vi "loadSchedule.vi"() -> ()   [LabVIEW 2012]
uses:
  <vilib>/Utility/NIReport.llb/NI_report.lvclass
  <vilib>/addons/database/Auxilliary.llb/DB Tools Cursor Type.ctl
  <vilib>/addons/_office/_exclsub.llb/font.ctl
  <vilib>/addons/_office/excel.llb/Excel Get Data (str).vi
  <vilib>/addons/database/Connection.llb/DB Tools Open Connec (Path).vi
  <vilib>/addons/database/Connection.llb/Conn Execute.vi
  <vilib>/addons/database/Recordset.llb/Rec Fetch Recordset Data (R).vi
  <vilib>/addons/database/Recordset.llb/Rec Destroy - Connection.vi
  <vilib>/addons/database/_DB Variant To Data/Database Variant To Data.xnode
  <vilib>/Utility/NIReport.llb/Excel/NI_Excel.lvclass
  <vilib>/addons/_office/NI_ReportGenerationToolkit.lvlib
  <vilib>/addons/database/NI_Database_API.lvlib
panel:
  out "spreadsheet string":string
  in  "start (0, 0) 4":cluster{"start row":i32, "start column":i32}
  out "ExcelRow":i32
  out "output cluster":cluster{"start row":i32, "start column":i32}
  in  "start (0, 0) 3":cluster{"start row":i32, "start column":i32}
  out "concatenated string":string
  in  "template (empty) 2":path=path "O:/m100schedule/history/112199MT人力配置AT機台排程.xls"
  out "error out 4":errorcluster
  out "array":string[][](array[string])
  in  "start (0, 0) 2":cluster{"start row":i32, "start column":i32}
  out "data":string
  in  "template (empty)":path=path "O:/m100schedule/history/m100-schedule temp.xls"
  in  "start (0, 0)":cluster{"start row":i32, "start column":i32}
  out "x+y":i32
  out "row":i32
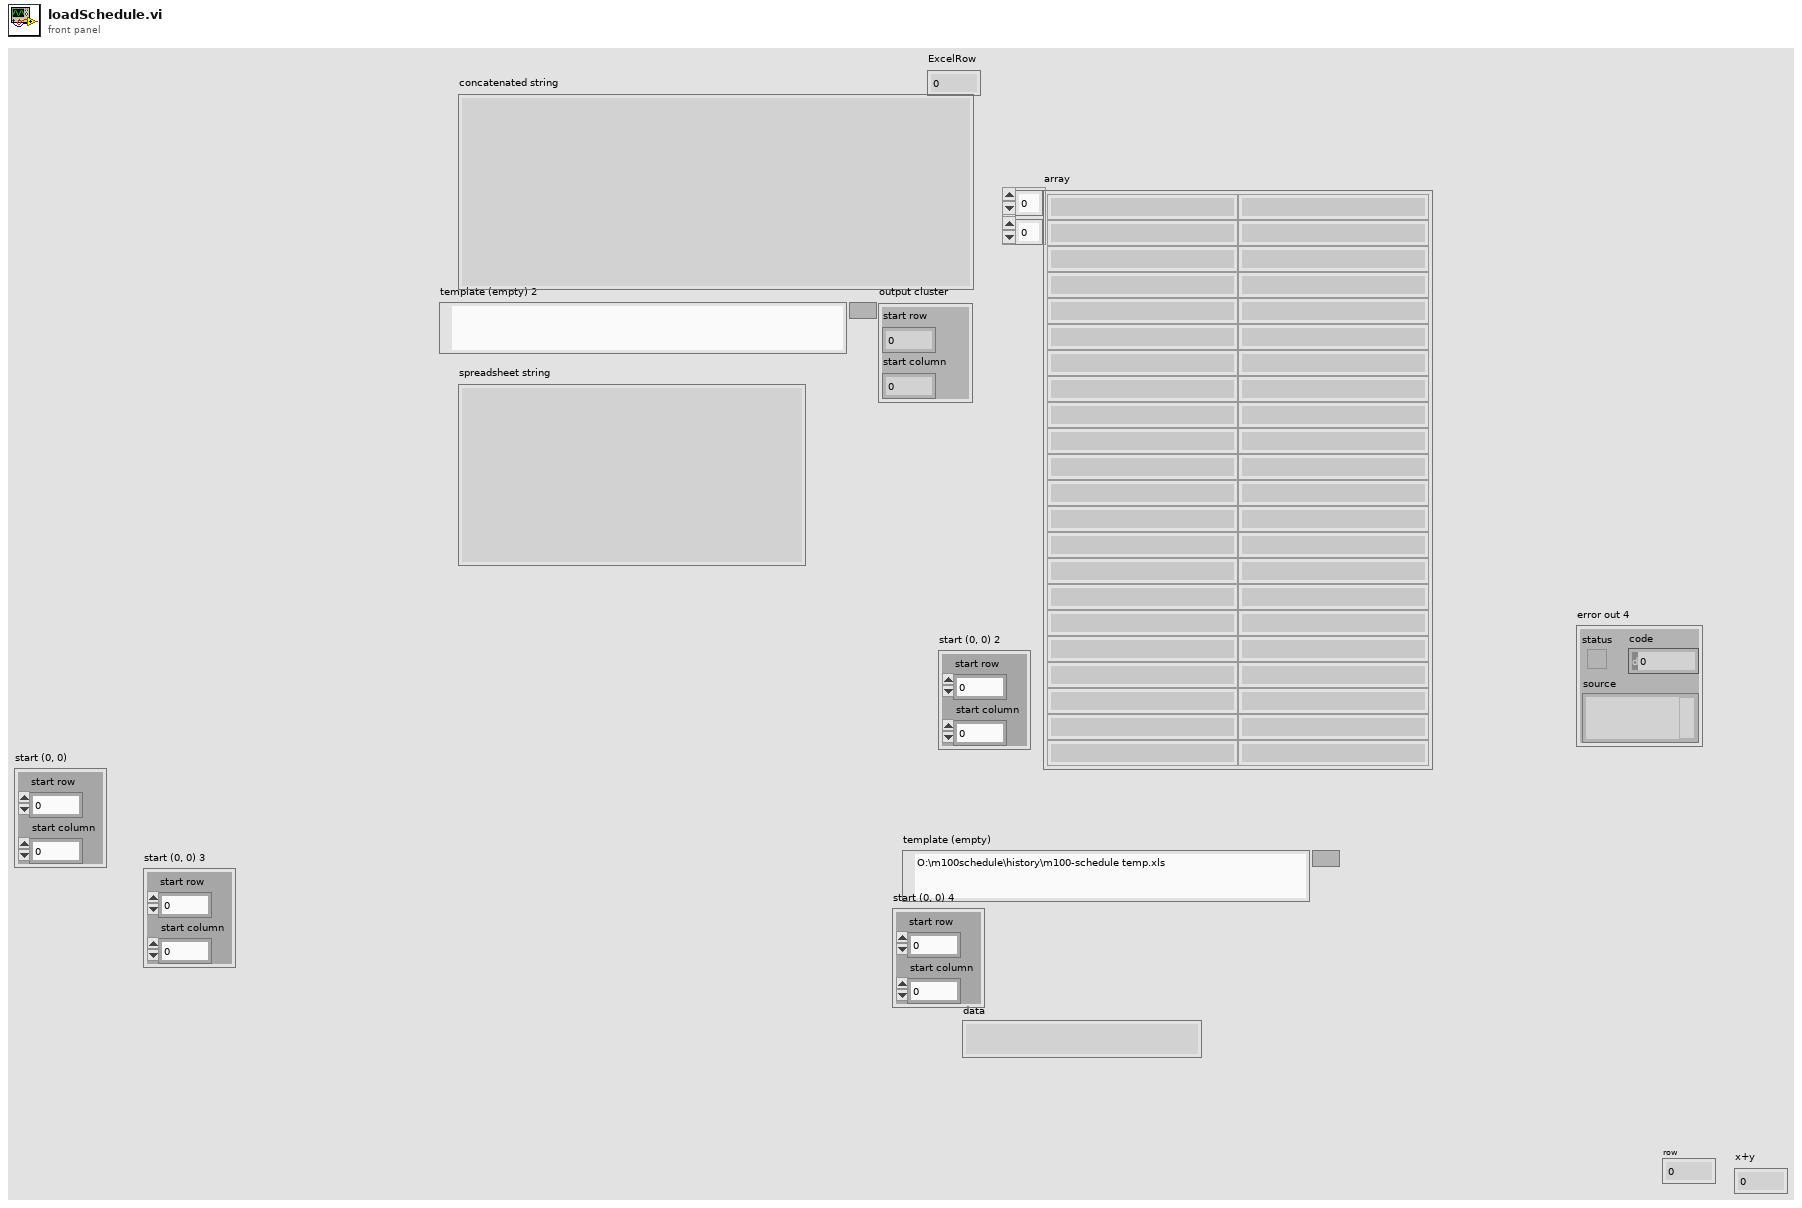
[diagram p1: front panel]
types:
  T1 = enum16{"Standard Report", "HTML", "Word", "Excel"}
  T2 = typedef "NI_Database_API.lvlib/DB Tools Cursor Type.ctl" = enum16{"forward-only", "keyset", "dynamic", "static"}
  T3 = typedef "NI_ReportGenerationToolkit.lvlib/font.ctl" = cluster{"font name":string, "font size":dbl, "bold":u16, "italic":u16, "underline":u16, "strike through":u16, "font color":u32}
  T4 = cluster{"on/off":bool, "weight":i32, "color":u32}
  T5 = typedef "NI_Database_API.lvlib/Conn ObjectReference.ctl" = refnum<k1>
  T6 = typedef "NI_Database_API.lvlib/Rec ObjectReference.ctl" = refnum<k1>
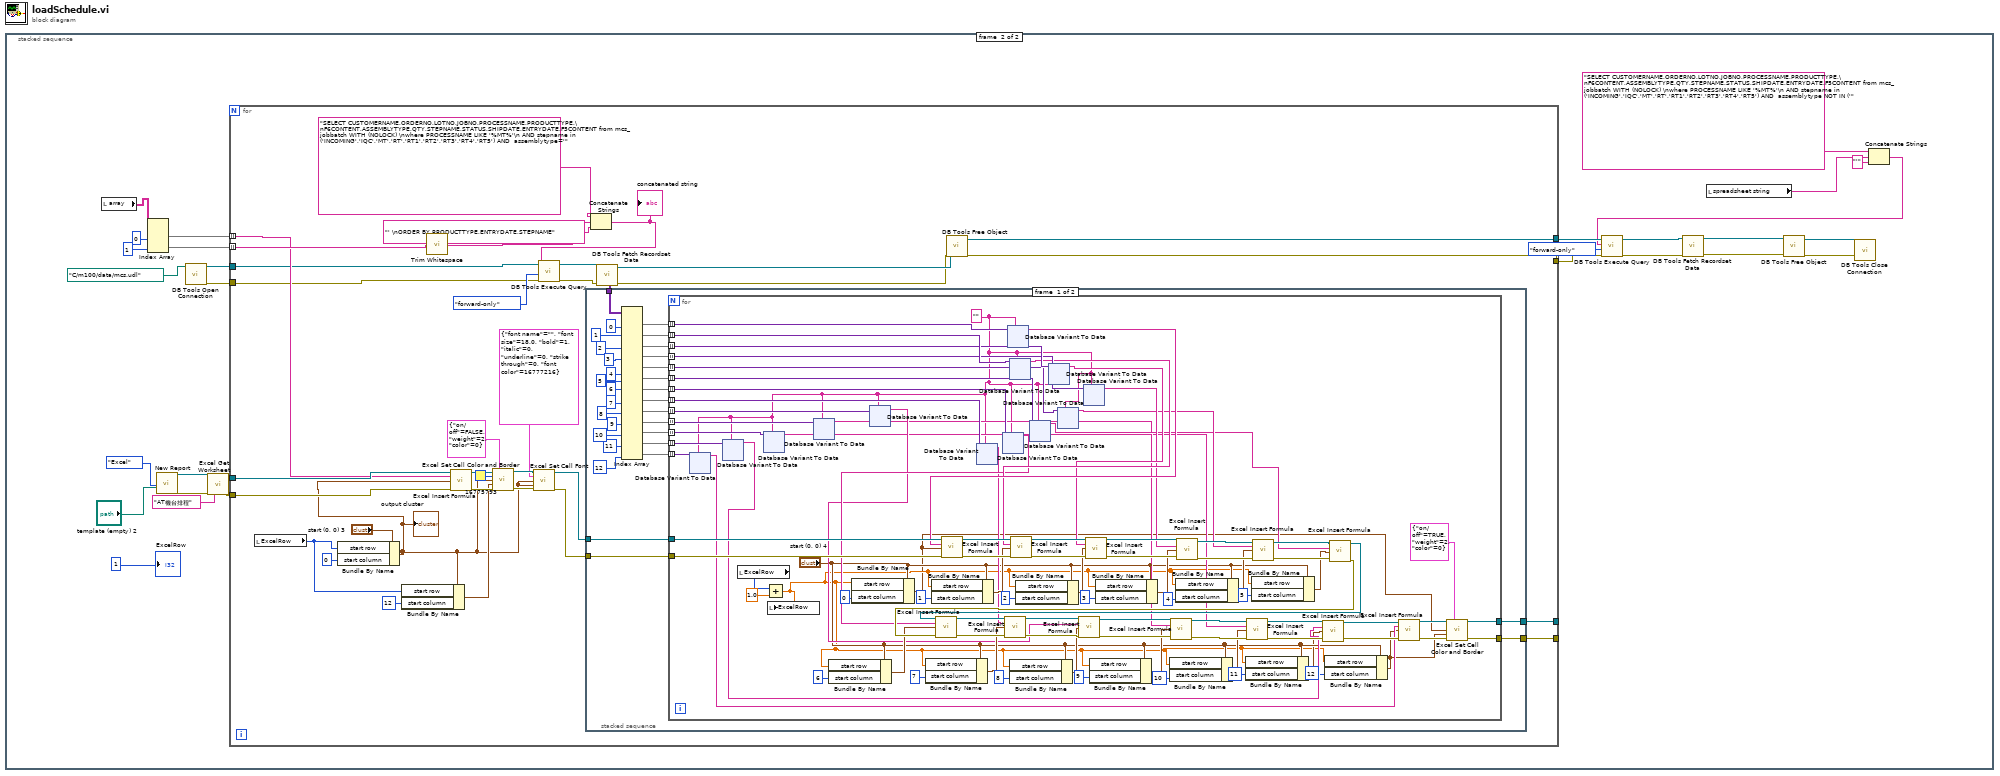
[diagram p0: block diagram]
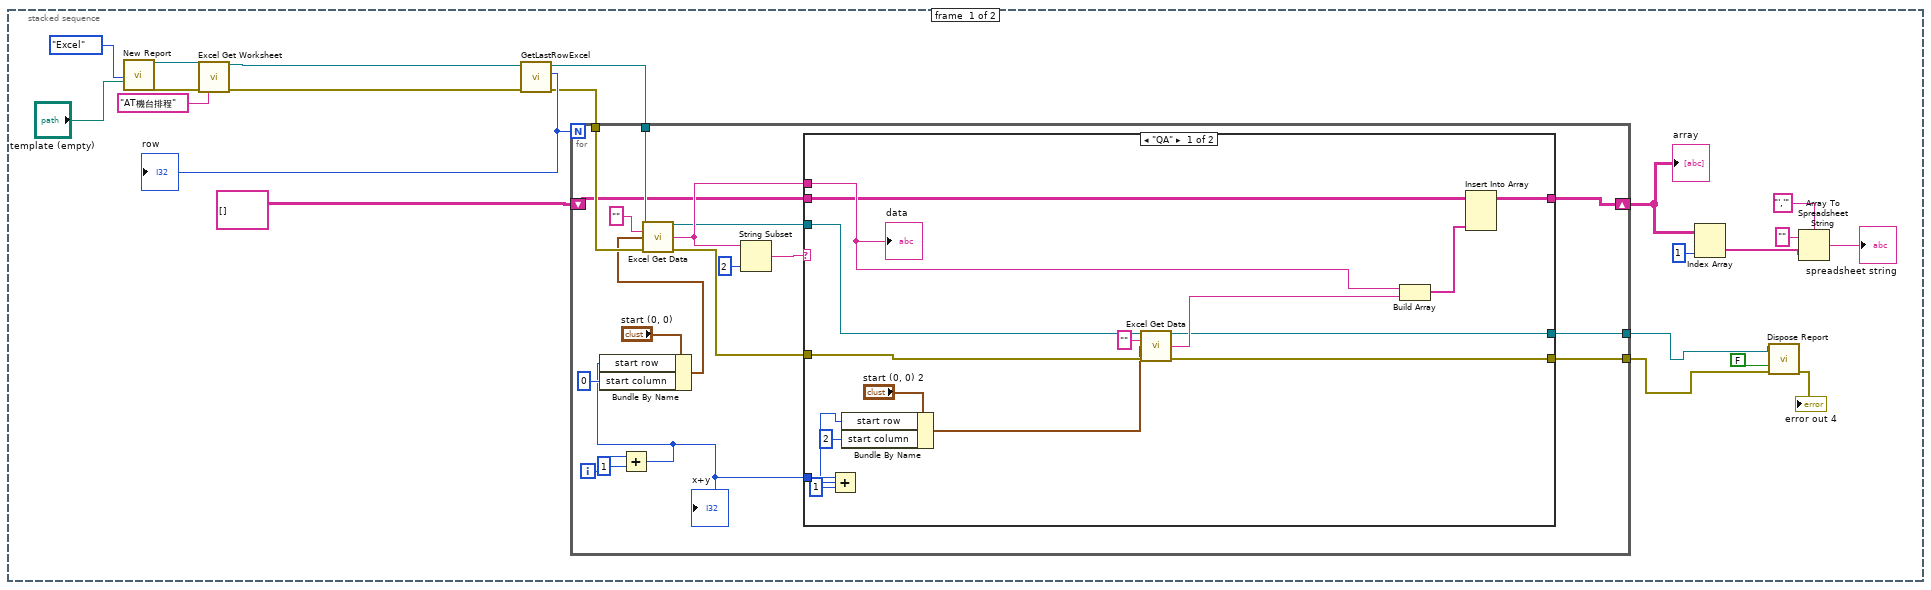
[diagram p2: hidden frame]
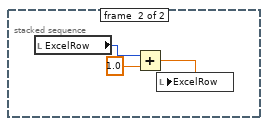
[diagram p4: hidden frame]
diagram:
  n1 = stacked-sequence {
    frame #0 {
      n2 = call <vilib>:"New Report.vi"("report type"=T1."Excel" ("Report Type"), "template (empty)"="template (empty)") -> ("report out"=w20:refnum<class "NI_report.lvclass">, "error out"=w19:errorcluster)  [unwired: 12 in]
      n3 = call <vilib>:"Excel Get Worksheet.vi"("report in"=w20, "error in (no error)"=w19, "name (\"\")"="AT機台排程" ("name (\"\")")) -> ("report out"=w18:refnum<class "NI_report.lvclass">, "error out"=w17:errorcluster)  [unwired: 11 in]
      n4 = call "GetLastRowExcel.vi"("error in (no error)"=w17, "report in"=w18) -> ("error out"=w13:errorcluster, "row"=w16:i32, "report out"=w12:refnum<class "NI_report.lvclass">)  [unwired: 7 in]
      "row" <- w16
      n5 = for {
        N: w16 -> [_]
        tunnel: w12 -> [w39]
        tunnel: w13 -> [w38]
        shift-right: [w27] -> w3
        shift-left: string[][] [] ("array") -> [w28]
        tunnel: [w23] -> w8
        tunnel: [w22] -> w7
        i -> [w34]
        n6 = Add(x=w34, y=1) -> (x+y=w24:i32)
        "x+y" <- w24
        n7 = Bundle By Name(cluster="start (0, 0)", "start row"=w24, "start column"=0) -> (w35:cluster{"start row":i32, "start column":i32})
        n8 = call-poly <vilib>:"Excel Get Data.vi"("report in"=w39, "data type"="", "start (0, 0)"=w35, "error in (no error)"=w38) -> ("report out"=w26:refnum<class "NI_report.lvclass">, "data"=w30:string, "error out"=w25:errorcluster)  [unwired: 9 in]
        n9 = String Subset(string=w30, length (rest)=2 ("length (rest)")) -> (substring=w31:string)  [unwired: 1 in]
        n10 = case shown="\"QA\"" w31 {
          tunnel: w30 -> [w55 _]
          tunnel: w28 -> [w52 w58]
          tunnel: [w53 w58] -> w27
          tunnel: w26 -> [w51 w57]
          tunnel: w25 -> [w50 w56]
          tunnel: w24 -> [w45 _]
          tunnel: [w41 w57] -> w23
          tunnel: [w40 w56] -> w22
          frame "QA" {
            n11 = Add(x=w45, y=1) -> (x+y=w43:i32)
            n12 = Bundle By Name(cluster="start (0, 0) 2", "start row"=w43, "start column"=2) -> (w48:cluster{"start row":i32, "start column":i32})
            n13 = call-poly <vilib>:"Excel Get Data.vi"("report in"=w51, "data type"="", "start (0, 0)"=w48, "error in (no error)"=w50) -> ("report out"=w41:refnum<class "NI_report.lvclass">, "data"=w42:string, "error out"=w40:errorcluster)  [unwired: 9 in]
            n14 = Build Array(w55, w42) -> (w54:string[])
            n15 = Insert Into Array(array=w52, new element=w54) -> (w53:string[][])  [unwired: 2 in]
            "data" <- w55
          }
          frame Default {
          }
        }
      }
      "array" <- w3
      n16 = Index Array(array=w3, index (col)=1 ("disabled index (col)")) -> (element=w1:string[])  [unwired: 1 in]
      n17 = call-dynamic "Dispose Report.vi"("report in"=w8, "save changes? (F)"=FALSE, "error in (no error)"=w7) -> ("error out"=→"error out 4":errorcluster)  [unwired: 12 in]
      n18 = Array To Spreadsheet String(delimiter (Tab)="','", array=w1, 3:"" ("format string")) -> (spreadsheet string=→"spreadsheet string":string)
    }
    frame #1 {
      n19 = local read "array"() -> (w82:string[][])
      n20 = Index Array(array=w82, index (col) #1=0 ("disabled index (col)"), index (col) #2=1 ("index (col)")) -> (element #1=w81:string[], element #2=w78:string[])  [unwired: 2 in]
      n21 = call <vilib>:"New Report.vi"("report type"=T1."Excel" ("Report Type"), "template (empty)"="template (empty) 2") -> ("report out"=w86:refnum<class "NI_report.lvclass">, "error out"=w85:errorcluster)  [unwired: 12 in]
      n22 = call-poly <vilib>:"DB Tools Open Connection.vi"("connection information"=path "C:/m100/data/mcs.udl") -> ("error out"=w72:errorcluster, "connection reference"=w73:T5)  [unwired: 7 in]
      n23 = call <vilib>:"Excel Get Worksheet.vi"("report in"=w86, "error in (no error)"=w85, "name (\"\")"="AT機台排程" ("name (\"\")")) -> ("report out"=w77:refnum<class "NI_report.lvclass">, "error out"=w76:errorcluster)  [unwired: 11 in]
      n24 = for {
        tunnel: w81 -> [w109] mode=indexing
        tunnel: w78 -> [w114] mode=indexing
        tunnel: w77 -> [w111]
        tunnel: w76 -> [w110]
        tunnel: [w93] -> _
        tunnel: [w92] -> _
        tunnel: w73 -> [w91]
        tunnel: w72 -> [w90]
        tunnel: [w89] -> w71
        tunnel: [w88] -> w70
        n25 = local read "ExcelRow"() -> (w102:i32)
        n26 = Bundle By Name(cluster="start (0, 0) 3", "start row"=w102, "start column"=0) -> (w95:cluster{"start row":i32, "start column":i32})
        "output cluster" <- w95
        n27 = Bundle By Name(cluster=w95, "start row"=w102, "start column"=12) -> (w100:cluster{"start row":i32, "start column":i32})
        n28 = call <vilib>:"Trim Whitespace.vi"("string"=w114) -> ("trimmed string"=w113:string)  [unwired: 1 in]
        n29 = call <vilib>:"Excel Insert Formula.vi"("report in"=w111, "formula"=w109, "start (0, 0)"=w95, "error in (no error)"=w110) -> ("report out"=w106:refnum<class "NI_report.lvclass">, "error out"=w105:errorcluster)  [unwired: 10 in]
        n30 = call <vilib>:"Excel Set Cell Color and Border.vi"("report in"=w106, "inside border"=T4 {"on/off"=FALSE, "weight"=2, "color"=0}, "background color (w)"=u32 16775793, "start (-1, -1)"=w95, "end (-1, -1)"=w100, "error in (no error)"=w105) -> ("report out"=w99:refnum<class "NI_report.lvclass">, "error out"=w98:errorcluster)  [unwired: 8 in]
        n31 = call <vilib>:"Excel Set Cell Font.vi"("report in"=w99, "font"=T3 {"font name"="", "font size"=18.0, "bold"=1, "italic"=0, "underline"=0, "strike through"=0, "font color"=16777216}, "start (-1, -1)"=w95, "end (-1, -1)"=w95, "error in (no error)"=w98) -> ("report out"=w97:refnum<class "NI_report.lvclass">, "error out"=w96:errorcluster)  [unwired: 9 in]
        n32 = Concatenate Strings("SELECT CUSTOMERNAME,ORDERNO,LOTNO,JOBNO,PROCESSNAME,PRODUCTTYPE,\nF6CONTENT,ASSEMBLYTYPE,QTY,STEPNAME,STATUS,SHIPDATE,ENTRYDATE,F5CONTENT from mcs_jobbatch WITH (NOLOCK) \nwhere PROCESSNAME LIKE '%MT%'\n AND stepname in ('INCOMING','IQC','MT','RT','RT1','RT2','RT3','RT4','RT5') AND  assemblytype='" ("SQL query"), w113, "' \nORDER BY PRODUCTTYPE,ENTRYDATE,STEPNAME" ("string")) -> (w116:string)
        "concatenated string" <- w116
        n33 = call-poly <vilib>:"DB Tools Execute Query.vi"("error in (no error)"=w90, "cursor type"=DB_Tools_Cursor_Type."forward-only", "SQL query"=w116, "connection reference"=w91) -> ("error out"=w120:errorcluster, "recordset reference"=w122:T6)  [unwired: 4 in]
        n34 = call-poly <vilib>:"DB Tools Fetch Recordset Data.vi"("error in (no error)"=w120, "recordset reference"=w122) -> ("error out"=w119:errorcluster, "recordset data"=w112:variant[][], "recordset reference out"=w121:T6)  [unwired: 3 in]
        n35 = stacked-sequence {
          tunnel: w112 -> [w153 _]
          tunnel: w97 -> [w136 _]
          tunnel: w96 -> [w135 _]
          tunnel: [w124 _] -> w93
          tunnel: [w123 _] -> w92
          frame #0 {
            n36 = Index Array(array=w153, index (col) #1=0 ("disabled index (col)"), index (col) #2=1 ("index (col)"), index (col) #3=2 ("index (col)"), index (col) #4=3 ("index (col)"), index (col) #5=4 ("index (col)"), index (col) #6=5 ("index (col)"), index (col) #7=6 ("index (col)"), index (col) #8=7 ("index (col)"), index (col) #9=8 ("index (col)"), index (col) #10=9 ("index (col)"), index (col) #11=10 ("index (col)"), index (col) #12=11 ("index (col)"), index (col) #13=12 ("index (col)")) -> (element #1=w144:variant[], element #2=w143:variant[], element #3=w142:variant[], element #4=w141:variant[], element #5=w140:variant[], element #6=w139:variant[], element #7=w138:variant[], element #8=w137:variant[], element #9=w131:variant[], element #10=w130:variant[], element #11=w129:variant[], element #12=w127:variant[], element #13=w125:variant[])  [unwired: 13 in]
            n37 = for {
              tunnel: w144 -> [w241] mode=indexing
              tunnel: w143 -> [w240] mode=indexing
              tunnel: w142 -> [w239] mode=indexing
              tunnel: w141 -> [w238] mode=indexing
              tunnel: w140 -> [w237] mode=indexing
              tunnel: w139 -> [w236] mode=indexing
              tunnel: w138 -> [w235] mode=indexing
              tunnel: w137 -> [w234] mode=indexing
              tunnel: w136 -> [w233]
              tunnel: w135 -> [w232]
              tunnel: w131 -> [w177] mode=indexing
              tunnel: w130 -> [w176] mode=indexing
              tunnel: w129 -> [w175] mode=indexing
              tunnel: w127 -> [w171] mode=indexing
              tunnel: w125 -> [w169] mode=indexing
              tunnel: [w155] -> w124
              tunnel: [w154] -> w123
              w168 = ""
              n38 = xnode "Database Variant To Data"("database variant"=w169, "type"=w168) -> ("data"=w161:string)  [unwired: 1 in, 1 out]
              n39 = xnode "Database Variant To Data"("database variant"=w171, "type"=w168) -> ("data"=w170:string)  [unwired: 1 in, 1 out]
              n40 = local read "ExcelRow"() -> (w229:i32)
              n41 = xnode "Database Variant To Data"("database variant"=w175, "type"=w168) -> ("data"=w172:string)  [unwired: 1 in, 1 out]
              n42 = Add(x=w229, y=1.0) -> (x+y=w165:dbl)
              n43 = local write "ExcelRow"(w165) -> ()
              n44 = xnode "Database Variant To Data"("database variant"=w176, "type"=w168) -> ("data"=w173:string)  [unwired: 1 in, 1 out]
              n45 = Bundle By Name(cluster="start (0, 0) 4", "start row"=w165, "start column"=6) -> (w180:cluster{"start row":i32, "start column":i32})
              n46 = Bundle By Name(cluster="start (0, 0) 4", "start row"=w165, "start column"=0) -> (w157:cluster{"start row":i32, "start column":i32})
              n47 = xnode "Database Variant To Data"("database variant"=w177, "type"=w168) -> ("data"=w174:string)  [unwired: 1 in, 1 out]
              n48 = Bundle By Name(cluster="start (0, 0) 4", "start row"=w165, "start column"=7) -> (w199:cluster{"start row":i32, "start column":i32})
              n49 = Bundle By Name(cluster="start (0, 0) 4", "start row"=w165, "start column"=1) -> (w223:cluster{"start row":i32, "start column":i32})
              n50 = xnode "Database Variant To Data"("database variant"=w234, "type"=w168) -> ("data"=w178:string)  [unwired: 1 in, 1 out]
              n51 = xnode "Database Variant To Data"("database variant"=w235, "type"=w168) -> ("data"=w179:string)  [unwired: 1 in, 1 out]
              n52 = xnode "Database Variant To Data"("database variant"=w241, "type"=w168) -> ("data"=w231:string)  [unwired: 1 in, 1 out]
              n53 = call <vilib>:"Excel Insert Formula.vi"("report in"=w233, "formula"=w231, "start (0, 0)"=w157, "error in (no error)"=w232) -> ("report out"=w226:refnum<class "NI_report.lvclass">, "error out"=w225:errorcluster)  [unwired: 10 in]
              n54 = xnode "Database Variant To Data"("database variant"=w240, "type"=w168) -> ("data"=w224:string)  [unwired: 1 in, 1 out]
              n55 = Bundle By Name(cluster="start (0, 0) 4", "start row"=w165, "start column"=8) -> (w195:cluster{"start row":i32, "start column":i32})
              n56 = call <vilib>:"Excel Insert Formula.vi"("report in"=w226, "formula"=w224, "start (0, 0)"=w223, "error in (no error)"=w225) -> ("report out"=w221:refnum<class "NI_report.lvclass">, "error out"=w220:errorcluster)  [unwired: 10 in]
              n57 = Bundle By Name(cluster="start (0, 0) 4", "start row"=w165, "start column"=2) -> (w219:cluster{"start row":i32, "start column":i32})
              n58 = xnode "Database Variant To Data"("database variant"=w236, "type"=w168) -> ("data"=w203:string)  [unwired: 1 in, 1 out]
              n59 = xnode "Database Variant To Data"("database variant"=w239, "type"=w168) -> ("data"=w218:string)  [unwired: 1 in, 1 out]
              n60 = xnode "Database Variant To Data"("database variant"=w237, "type"=w168) -> ("data"=w208:string)  [unwired: 1 in, 1 out]
              n61 = xnode "Database Variant To Data"("database variant"=w238, "type"=w168) -> ("data"=w213:string)  [unwired: 1 in, 1 out]
              n62 = call <vilib>:"Excel Insert Formula.vi"("report in"=w221, "formula"=w218, "start (0, 0)"=w219, "error in (no error)"=w220) -> ("report out"=w216:refnum<class "NI_report.lvclass">, "error out"=w215:errorcluster)  [unwired: 10 in]
              n63 = Bundle By Name(cluster="start (0, 0) 4", "start row"=w165, "start column"=9) -> (w191:cluster{"start row":i32, "start column":i32})
              n64 = Bundle By Name(cluster="start (0, 0) 4", "start row"=w165, "start column"=3) -> (w214:cluster{"start row":i32, "start column":i32})
              n65 = Bundle By Name(cluster="start (0, 0) 4", "start row"=w165, "start column"=10) -> (w187:cluster{"start row":i32, "start column":i32})
              n66 = Bundle By Name(cluster="start (0, 0) 4", "start row"=w165, "start column"=4) -> (w209:cluster{"start row":i32, "start column":i32})
              n67 = call <vilib>:"Excel Insert Formula.vi"("report in"=w216, "formula"=w213, "start (0, 0)"=w214, "error in (no error)"=w215) -> ("report out"=w211:refnum<class "NI_report.lvclass">, "error out"=w210:errorcluster)  [unwired: 10 in]
              n68 = Bundle By Name(cluster="start (0, 0) 4", "start row"=w165, "start column"=11) -> (w166:cluster{"start row":i32, "start column":i32})
              n69 = Bundle By Name(cluster="start (0, 0) 4", "start row"=w165, "start column"=5) -> (w204:cluster{"start row":i32, "start column":i32})
              n70 = call <vilib>:"Excel Insert Formula.vi"("report in"=w211, "formula"=w208, "start (0, 0)"=w209, "error in (no error)"=w210) -> ("report out"=w206:refnum<class "NI_report.lvclass">, "error out"=w205:errorcluster)  [unwired: 10 in]
              n71 = Bundle By Name(cluster="start (0, 0) 4", "start row"=w165, "start column"=12) -> (w156:cluster{"start row":i32, "start column":i32})
              n72 = call <vilib>:"Excel Insert Formula.vi"("report in"=w206, "formula"=w203, "start (0, 0)"=w204, "error in (no error)"=w205) -> ("report out"=w183:refnum<class "NI_report.lvclass">, "error out"=w182:errorcluster)  [unwired: 10 in]
              n73 = call <vilib>:"Excel Insert Formula.vi"("report in"=w183, "formula"=w179, "start (0, 0)"=w180, "error in (no error)"=w182) -> ("report out"=w201:refnum<class "NI_report.lvclass">, "error out"=w200:errorcluster)  [unwired: 10 in]
              n74 = call <vilib>:"Excel Insert Formula.vi"("report in"=w201, "formula"=w178, "start (0, 0)"=w199, "error in (no error)"=w200) -> ("report out"=w197:refnum<class "NI_report.lvclass">, "error out"=w196:errorcluster)  [unwired: 10 in]
              n75 = call <vilib>:"Excel Insert Formula.vi"("report in"=w197, "formula"=w174, "start (0, 0)"=w195, "error in (no error)"=w196) -> ("report out"=w193:refnum<class "NI_report.lvclass">, "error out"=w192:errorcluster)  [unwired: 10 in]
              n76 = call <vilib>:"Excel Insert Formula.vi"("report in"=w193, "formula"=w173, "start (0, 0)"=w191, "error in (no error)"=w192) -> ("report out"=w189:refnum<class "NI_report.lvclass">, "error out"=w188:errorcluster)  [unwired: 10 in]
              n77 = call <vilib>:"Excel Insert Formula.vi"("report in"=w189, "formula"=w172, "start (0, 0)"=w187, "error in (no error)"=w188) -> ("report out"=w185:refnum<class "NI_report.lvclass">, "error out"=w184:errorcluster)  [unwired: 10 in]
              n78 = call <vilib>:"Excel Insert Formula.vi"("report in"=w185, "formula"=w170, "start (0, 0)"=w166, "error in (no error)"=w184) -> ("report out"=w162:refnum<class "NI_report.lvclass">, "error out"=w163:errorcluster)  [unwired: 10 in]
              n79 = call <vilib>:"Excel Insert Formula.vi"("report in"=w162, "formula"=w161, "start (0, 0)"=w156, "error in (no error)"=w163) -> ("report out"=w160:refnum<class "NI_report.lvclass">, "error out"=w159:errorcluster)  [unwired: 10 in]
              n80 = call <vilib>:"Excel Set Cell Color and Border.vi"("report in"=w160, "inside border"=T4 {"on/off"=TRUE, "weight"=2, "color"=0}, "start (-1, -1)"=w157, "end (-1, -1)"=w156, "error in (no error)"=w159) -> ("report out"=w155:refnum<class "NI_report.lvclass">, "error out"=w154:errorcluster)  [unwired: 9 in]
            }
          }
          frame #1 {
            n81 = local read "ExcelRow"() -> (w659:i32)
            n82 = Add(x=w659, y=1.0) -> (x+y=w658:dbl)
            n83 = local write "ExcelRow"(w658) -> ()
          }
        }
        n84 = call-poly <vilib>:"DB Tools Free Object.vi"("error in (no error)"=w119, "recordset reference"=w121) -> ("error out"=w88:errorcluster, "connection reference"=w89:T5)  [unwired: 8 in]
      }
      n85 = local read "spreadsheet string"() -> (w61:string)
      n86 = Concatenate Strings("SELECT CUSTOMERNAME,ORDERNO,LOTNO,JOBNO,PROCESSNAME,PRODUCTTYPE,\nF6CONTENT,ASSEMBLYTYPE,QTY,STEPNAME,STATUS,SHIPDATE,ENTRYDATE,F5CONTENT from mcs_jobbatch WITH (NOLOCK) \nwhere PROCESSNAME LIKE '%MT%'\n AND stepname in ('INCOMING','IQC','MT','RT','RT1','RT2','RT3','RT4','RT5') AND  assemblytype NOT IN ('" ("SQL query"), w61, "'" ("string")) -> (w59:string)
      n87 = call-poly <vilib>:"DB Tools Execute Query.vi"("error in (no error)"=w70, "cursor type"=DB_Tools_Cursor_Type."forward-only", "SQL query"=w59, "connection reference"=w71) -> ("error out"=w67:errorcluster, "recordset reference"=w69:T6)  [unwired: 4 in]
      n88 = call-poly <vilib>:"DB Tools Fetch Recordset Data.vi"("error in (no error)"=w67, "recordset reference"=w69) -> ("error out"=w66:errorcluster, "recordset reference out"=w68:T6)  [unwired: 3 in, 1 out]
      n89 = call-poly <vilib>:"DB Tools Free Object.vi"("error in (no error)"=w66, "recordset reference"=w68) -> ("error out"=w65:errorcluster, "connection reference"=w64:T5)  [unwired: 8 in]
      n90 = call <vilib>:"DB Tools Close Connection.vi"("error in (no error)"=w65, "connection reference"=w64) -> ()  [unwired: 5 in, 1 out]
      "ExcelRow" <- 1
    }
  }
